vi "Center of mass in array range.vi"(9 "1/2 Width  (pixels)":i32, 11 "Data":dbl[](array[numeric])) -> (1 "Average value":dbl, 3 "Center Index":dbl)   [LabVIEW 2013]
doc: "Determines the center of mass about a point (max) in an array"
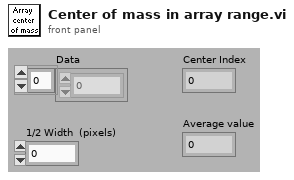
[diagram p1: front panel]
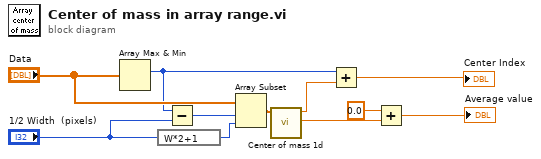
[diagram p0: block diagram]
diagram:
  n1 = Array Max & Min(array="Data") -> (max index (indices)=w4:i32)  [unwired: 3 out]
  n2 = expression code="W*2+1"("1/2 Width  (pixels)") -> (w9:i32)
  n3 = Subtract(x=w4, y="1/2 Width  (pixels)") -> (x-y=w8:i32)
  n4 = Array Subset(array="Data", index=w8, length=w9) -> (w10:dbl[])
  n5 = call "Center of mass 1d.vi"("Data in"=w10) -> ("Average value"=w6:dbl, "Center of mass offset"=w3:dbl)  [unwired: 9 out]
  n6 = Add(x=w4, y=w3) -> (x+y=→"Center Index":dbl)
  n7 = Add(x=0.0, y=w6) -> (x+y=→"Average value":dbl)
